vi "CAEN_HVChannel.contents.vi"   [LabVIEW 2014, in "CAEN_HVChannel.lvlib"]
doc: "This VI contains all dynamically called VIs. To be used in build specifications."
uses:
  CAEN_HVChannel.lvlib
panel:
  # "Refer to blockdiagram for content VIs."
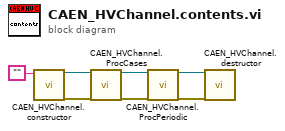
[diagram p0: block diagram]
diagram:
  n1 = call "CAEN_HVChannel.constructor.vi"("name"="") -> ("i ref out"=w5:refnum<vi>, "error out"=w4:errorcluster)  [unwired: 16 in, 1 out]
  n2 = call "CAEN_HVChannel.ProcCases.vi"("i ref in"=w5, "error in (no error)"=w4) -> ("i ref out"=w6:refnum<vi>, "error out"=w3:errorcluster)  [unwired: 15 in, 1 out]
  n3 = call "CAEN_HVChannel.ProcPeriodic.vi"("i ref in"=w6, "error in (no error)"=w3) -> ("i ref out"=w7:refnum<vi>, "error out"=w2:errorcluster)  [unwired: 15 in, 1 out]
  n4 = call "CAEN_HVChannel.destructor.vi"("i ref in"=w7, "error in(no error)"=w2) -> ()  [unwired: 17 in, 1 out]
